vi "Main Globals.vi"() -> ()   [LabVIEW 2018]
panel:
  in  "Pause Log":bool
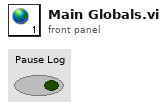
[diagram p1: front panel]
diagram:
